vi "blob write.vi"(7 "iOffset":i32, 8 "error in (no error)":errorcluster, 9 "n":i32, 10 "z":u32, 11 "para0":dbl) -> (0 "error out":errorcluster, 2 "function return":i32, 3 "para0 out":dbl)   [LabVIEW 2020, in "sqlite3.lvlib"]
uses:
  sqlite3.lvlib
  errstr.vi
  bin/sqlite3_64.dll
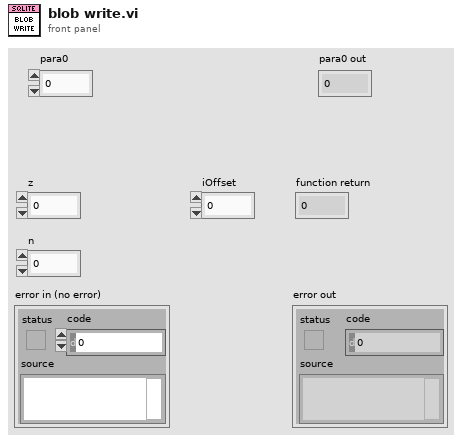
[diagram p1: front panel]
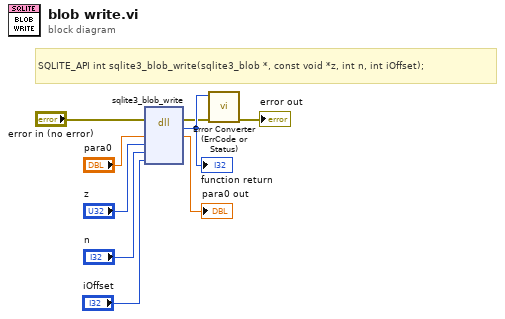
[diagram p0: block diagram]
diagram:
  # "SQLITE_API int sqlite3_blob_write(sqlite3_blob *, const void *z, int n, int iOffset);"
  n1 = dll-call lib="C:/Users/Fred.Guo/Desktop/Database-configuration/externals/sqlite3/Source/bin/sqlite3_*.*" fn="sqlite3_blob_write"(error in="error in (no error)", "para0"="para0", "z"="z", "n"="n", "iOffset"="iOffset") -> (error out=w2:errorcluster, w9:i32, "para0"=→"para0 out":dbl)  [unwired: 5 in, 1 out]
  "function return" <- w9
  n2 = call "Error Converter (ErrCode or Status).vi"("error in (no error)"=w2, "error code"=w9) -> ("error out"=→"error out":errorcluster)  [unwired: 9 in]
